vi "Weather Parse Test.vi"() -> ()   [LabVIEW 2020, in "CDM-Config.lvlib"] (continued)
             \"CMAS\"\n                    ],\n                    \"VTEC\": [\n                        \"/O.CON.KBUF.SC.Y.0098.251203T1200Z-251205T0300Z/\"\n                    ],\n                    \"eventEndingTime\": [\n                        \"2025-12-04T22:00:00-05:00\"\n                    ]\n                },\n                \"scope\": \"Public\",\n                \"code\": \"IPAWSv1.0\",\n                \"language\": \"en-US\",\n                \"web\": \"http://www.weather.gov\",\n                \"eventCode\": {\n                    \"SAME\": [\n                        \"NWS\"\n                    ],\n                    \"NationalWeatherService\": [\n                        \"SCY\"\n                    ]\n                }\n            }\n        },\n        {\n            \"id\": \"https://api.weather.gov/alerts/urn:oid:2.49.0.1.840.0.c02a5c0c1925cdd5918687c0525e8f8235dbd8da.001.1\",\n            \"type\": \"Feature\",\n            \"geometry\": null,\n            \"properties\": {\n                \"@id\": \"https://api.weather.gov/alerts/urn:oid:2.49.0.1.840.0.c02a5c0c1925cdd5918687c0525e8f8235dbd8da.001.1\",\n                \"@type\": \"wx:Alert\",\n                \"id\": \"urn:oid:2.49.0.1.840.0.c02a5c0c1925cdd5918687c0525e8f8235dbd8da.001.1\",\n                \"areaDesc\": \"Alger; Luce; Northern Schoolcraft\",\n                \"geocode\": {\n                    \"SAME\": [\n                        \"026003\",\n                        \"026095\",\n                        \"026153\"\n                    ],\n                    \"UGC\": [\n                        \"MIZ006\",\n                        \"MIZ007\",\n                        \"MIZ085\"\n                    ]\n                },\n                \"affectedZones\": [\n                    \"https://api.weather.gov/zones/forecast/MIZ006\",\n                    \"https://api.weather.gov/zones/forecast/MIZ007\",\n                    \"https://api.weather.gov/zones/forecast/MIZ085\"\n                ],\n                \"references\": [],\n                \"sent\": \"2025-12-03T03:02:00-05:00\",\n                \"effective\": \"2025-12-03T03:02:00-05:00\",\n                \"onset\": \"2025-12-03T07:00:00-05:00\",\n                \"expires\": \"2025-12-03T16:15:00-05:00\",\n                \"ends\": \"2025-12-04T07:00:00-05:00\",\n                \"status\": \"Actual\",\n                \"messageType\": \"Alert\",\n                \"category\": \"Met\",\n                \"severity\": \"Moderate\",\n                \"certainty\": \"Likely\",\n                \"urgency\": \"Expected\",\n                \"event\": \"Winter Weather Advisory\",\n                \"sender\": \"w-nws.webmaster@noaa.gov\",\n                \"senderName\": \"NWS Marquette MI\",\n                \"headline\": \"Winter Weather Advisory issued December 3 at 3:02AM EST until December 4 at 7:00AM EST by NWS Marquette MI\",\n                \"description\": \"* WHAT...Lake effect snow expected. Total snow accumulations between\\n3 and 7 inches. Winds gusting as high as 35 mph, highest along the\\nLake Superior shores.\\n\\n* WHERE...Alger, Luce, and Northern Schoolcraft Counties.\\n\\n* WHEN...From 7 AM this morning to 7 AM EST Thursday.\\n\\n* IMPACTS...Travel could be difficult. Areas of blowing snow could\\nsignificantly reduce visibility. The hazardous conditions could\\nimpact the Wednesday morning and evening commutes.\\n\\n* ADDITIONAL DETAILS...The southwest portions of Alger County such\\nas Chatham and Trenary will see snow accumulations of 2 inches or\\nless.\",\n                \"instruction\": \"Slow down and use caution while traveling.\\n\\nDuring lake effect snow, the weather can vary from bands of locally\\nheavy snow to dry weather just a few miles away. Visibilities can\\nalso vary greatly. Be prepared for rapid changes in weather,\\nvisibility, and road conditions.\",\n                \"response\": \"Execute\",\n                \"parameters\": {\n                    \"AWIPSidentifier\": [\n                        \"WSWMQT\"\n                    ],\n                    \"WMOidentifier\": [\n                        \"WWUS43 KMQT 030802\"\n                    ],\n                    \"NWSheadline\": [\n                        \"WINTER WEATHER ADVISORY IN EFFECT FROM 7 AM THIS MORNING TO 7 AM EST THURSDAY\"\n                    ],\n                    \"BLOCKCHANNEL\": [\n                        \"EAS\",\n                        \"NWEM\",\n                        \"CMAS\"\n                    ],\n                    \"VTEC\": [\n                        \"/O.NEW.KMQT.WW.Y.0035.251203T1200Z-251204T1200Z/\"\n                    ],\n                    \"eventEndingTime\": [\n                        \"2025-12-04T07:00:00-05:00\"\n                    ]\n                },\n                \"scope\": \"Public\",\n                \"code\": \"IPAWSv1.0\",\n                \"language\": \"en-US\",\n                \"web\": \"http://www.weather.gov\",\n                \"eventCode\": {\n                    \"SAME\": [\n                        \"NWS\"\n                    ],\n                    \"NationalWeatherService\": [\n                        \"WWY\"\n                    ]\n                }\n            }\n        },\n        {\n            \"id\": \"https://api.weather.gov/alerts/urn:oid:2.49.0.1.840.0.59f7e1922117cec0abab2205c7453e67e9856636.002.1\",\n            \"type\": \"Feature\",\n            \"geometry\": null,\n            \"properties\": {\n                \"@id\": \"https://api.weather.gov/alerts/urn:oid:2.49.0.1.840.0.59f7e1922117cec0abab2205c7453e67e9856636.002.1\",\n                \"@type\": \"wx:Alert\",\n                \"id\": \"urn:oid:2.49.0.1.840.0.59f7e1922117cec0abab2205c7453e67e9856636.002.1\",\n                \"areaDesc\": \"Sierra Madre Range; Snowy Range\",\n                \"geocode\": {\n                    \"SAME\": [\n                        \"056007\",\n                        \"056001\"\n                    ],\n                    \"UGC\": [\n                        \"WYZ112\",\n                        \"WYZ114\"\n                    ]\n                },\n                \"affectedZones\": [\n                    \"https://api.weather.gov/zones/forecast/WYZ112\",\n                    \"https://api.weather.gov/zones/forecast/WYZ114\"\n                ],\n                \"references\": [\n                    {\n                        \"@id\": \"https://api.weather.gov/alerts/urn:oid:2.49.0.1.840.0.87fb13f6ba1b004b93c1e82c033f30d580049308.002.1\",\n                        \"identifier\": \"urn:oid:2.49.0.1.840.0.87fb13f6ba1b004b93c1e82c033f30d580049308.002.1\",\n                        \"sender\": \"w-nws.webmaster@noaa.gov\",\n                        \"sent\": \"2025-12-02T14:13:00-07:00\"\n                    }\n                ],\n                \"sent\": \"2025-12-02T23:52:00-07:00\",\n                \"effective\": \"2025-12-02T23:52:00-07:00\",\n                \"onset\": \"2025-12-02T23:52:00-07:00\",\n                \"expires\": \"2025-12-03T11:00:00-07:00\",\n                \"ends\": \"2025-12-03T11:00:00-07:00\",\n                \"status\": \"Actual\",\n                \"messageType\": \"Update\",\n                \"category\": \"Met\",\n                \"severity\": \"Moderate\",\n                \"certainty\": \"Likely\",\n                \"urgency\": \"Expected\",\n                \"event\": \"Winter Weather Advisory\",\n                \"sender\": \"w-nws.webmaster@noaa.gov\",\n                \"senderName\": \"NWS Cheyenne WY\",\n                \"headline\": \"Winter Weather Advisory issued December 2 at 11:52PM MST until December 3 at 11:00AM MST by NWS Cheyenne WY\",\n                \"description\": \"* WHAT...Snow. Additional snow accumulations up to 3 inches.\\n\\n* WHERE...Sierra Madre Range and Snowy Range.\\n\\n* WHEN...Until 11 AM MST Wednesday.\\n\\n* IMPACTS...Outdoor recreation could become dangerous to those\\ncaught unprepared for hazardous winter conditions. Hunters,\\nhikers, and snowmobilers may become disoriented and lost due to\\nlow visibility in falling and blowing snow. Travel could be very\\ndifficult.\",\n                \"instruction\": \"Slow down and use caution while traveling. The latest road\\nconditions for the state you are calling from can be obtained by\\ncalling 5 1 1.\",\n                \"response\": \"Execute\",\n                \"parameters\": {\n                    \"AWIPSidentifier\": [\n                        \"WSWCYS\"\n                    ],\n                    \"WMOidentifier\": [\n                        \"WWUS45 KCYS 030652\"\n                    ],\n                    \"NWSheadline\": [\n                        \"WINTER WEATHER ADVISORY REMAINS IN EFFECT UNTIL 11 AM MST WEDNESDAY\"\n                    ],\n                    \"BLOCKCHANNEL\": [\n                        \"EAS\",\n                        \"NWEM\",\n                        \"CMAS\"\n                    ],\n                    \"VTEC\": [\n                        \"/O.CON.KCYS.WW.Y.0035.000000T0000Z-251203T1800Z/\"\n                    ],\n                    \"eventEndingTime\": [\n                        \"2025-12-03T11:00:00-07:00\"\n                    ],\n                    \"expiredReferences\": [\n                        \"w-nws.webmaster@noaa.gov,urn:oid:2.49.0.1.840.0.fecf578d7cc004b2e9035df7c924d23aa49b7b6f.001.1,2025-12-02T02:18:00-07:00 w-nws.webmaster@noaa.gov,urn:oid:2.49.0.1.840.0.569ad64d3405614b0a2aabc3905b3b5007dab878.001.1,2025-12-01T14:15:00-07:00 w-nws.webmaster@noaa.gov,urn:oid:2.49.0.1.840.0.9d0e156dd967b121facde90ef95bedbde49aa40d.001.1,2025-12-01T14:12:00-07:00\"\n                    ]\n                },\n                \"scope\": \"Public\",\n                \"code\": \"IPAWSv1.0\",\n                \"language\": \"en-US\",\n                \"web\": \"http://www.weather.gov\",\n                \"eventCode\": {\n                    \"SAME\": [\n                        \"NWS\"\n                    ],\n                    \"NationalWeatherService\": [\n                        \"WWY\"\n                    ]\n                }\n            }\n        },\n        {\n            \"id\": \"https://api.weather.gov/alerts/urn:oid:2.49.0.1.840.0.59f7e1922117cec0abab2205c7453e67e9856636.001.1\",\n            \"type\": \"Feature\",\n            \"geometry\": null,\n            \"properties\": {\n                \"@id\": \"https://api.weather.gov/alerts/urn:oid:2.49.0.1.840.0.59f7e1922117cec0abab2205c7453e67e9856636.001.1\",\n                \"@type\": \"wx:Alert\",\n                \"id\": \"urn:oid:2.49.0.1.840.0.59f7e1922117cec0abab2205c7453e67e9856636.001.1\",\n                \"areaDesc\": \"North Snowy Range Foothills; South Laramie Range\",\n                \"geocode\": {\n                    \"SAME\": [\n                        \"056001\",\n                        \"056007\",\n                        \"056021\"\n                    ],\n                    \"UGC\": [\n                        \"WYZ110\",\n                        \"WYZ116\"\n                    ]\n                },\n                \"affectedZones\": [\n                    \"https://api.weather.gov/zones/forecast/WYZ110\",\n                    \"https://api.weather.gov/zones/forecast/WYZ116\"\n                ],\n                \"references\": [\n                    {\n                        \"@id\": \"https://api.weather.gov/alerts/urn:oid:2.49.0.1.840.0.87fb13f6ba1b004b93c1e82c033f30d580049308.001.1\",\n                        \"identifier\": \"urn:oid:2.49.0.1.840.0.87fb13f6ba1b004b93c1e82c033f30d580049308.001.1\",\n                        \"sender\": \"w-nws.webmaster@noaa.gov\",\n                        \"sent\": \"2025-12-02T14:13:00-07:00\"\n                    }\n                ],\n                \"sent\": \"2025-12-02T23:52:00-07:00\",\n                \"effective\": \"2025-12-02T23:52:00-07:00\",\n                \"onset\": \"2025-12-02T23:52:00-07:00\",\n                \"expires\": \"2025-12-03T11:00:00-07:00\",\n                \"ends\": \"2025-12-03T11:00:00-07:00\",\n                \"status\": \"Actual\",\n                \"messageType\": \"Update\",\n                \"category\": \"Met\",\n                \"severity\": \"Moderate\",\n                \"certainty\": \"Likely\",\n                \"urgency\": \"Expected\",\n                \"event\": \"Winter Weather Advisory\",\n                \"sender\": \"w-nws.webmaster@noaa.gov\",\n                \"senderName\": \"NWS Cheyenne WY\",\n                \"headline\": \"Winter Weather Advisory issued December 2 at 11:52PM MST until December 3 at 11:00AM MST by NWS Cheyenne WY\",\n                \"description\": \"* WHAT...Snow. Additional snow accumulations up to two inches.\\n\\n* WHERE...South Laramie Range including the Interstate 80 Summit\\nbetween Cheyenne and Laramie, and North Snowy Range Foothills\\nincluding Arlington and Elk Mountain along Interstate 80.\\n\\n* WHEN...Until 11 AM MST Wednesday.\\n\\n* IMPACTS...Plan on slippery road conditions. The hazardous\\nconditions could impact the Wednesday morning commute.\",\n                \"instruction\": \"Slow down and use caution while traveling. The latest road\\nconditions for the state you are calling from can be obtained by\\ncalling 5 1 1.\",\n                \"response\": \"Execute\",\n                \"parameters\": {\n                    \"AWIPSidentifier\": [\n                        \"WSWCYS\"\n                    ],\n                    \"WMOidentifier\": [\n                        \"WWUS45 KCYS 030652\"\n                    ],\n                    \"NWSheadline\": [\n                        \"WINTER WEATHER ADVISORY REMAINS IN EFFECT UNTIL 11 AM MST WEDNESDAY\"\n                    ],\n                    \"BLOCKCHANNEL\": [\n                        \"EAS\",\n                        \"NWEM\",\n                        \"CMAS\"\n                    ],\n                    \"VTEC\": [\n                        \"/O.CON.KCYS.WW.Y.0035.000000T0000Z-251203T1800Z/\"\n                    ],\n                    \"eventEndingTime\": [\n                        \"2025-12-03T11:00:00-07:00\"\n                    ]\n                },\n                \"scope\": \"Public\",\n                \"code\": \"IPAWSv1.0\",\n                \"language\": \"en-US\",\n                \"web\": \"http://www.weather.gov\",\n                \"eventCode\": {\n                    \"SAME\": [\n                        \"NWS\"\n                    ],\n                    \"NationalWeatherService\": [\n                        \"WWY\"\n                    ]\n                }\n            }\n        },\n        {\n            \"id\": \"https://api.weather.gov/alerts/urn:oid:2.49.0.1.840.0.f60d42f0491b4e02db9492f5ccb8a64bf6617900.001.1\",\n            \"type\": \"Feature\",\n            \"geometry\": null,\n            \"properties\": {\n                \"@id\": \"https://api.weather.gov/alerts/urn:oid:2.49.0.1.840.0.f60d42f0491b4e02db9492f5ccb8a64bf6617900.001.1\",\n                \"@type\": \"wx:Alert\",\n                \"id\": \"urn:oid:2.49.0.1.840.0.f60d42f0491b4e02db9492f5ccb8a64bf6617900.001.1\",\n                \"areaDesc\": \"Chuuk Lagoon\",\n                \"geocode\": {\n                    \"SAME\": [\n                        \"064002\"\n                    ],\n                    \"UGC\": [\n                        \"FMZ023\"\n                    ]\n                },\n                \"affectedZones\": [\n                    \"https://api.weather.gov/zones/forecast/FMZ023\"\n                ],\n                \"references\": [],\n                \"sent\": \"2025-12-03T16:48:00+10:00\",\n                \"effective\": \"2025-12-03T16:48:00+10:00\",\n                \"onset\": \"2025-12-04T17:00:00+10:00\",\n                \"expires\": \"2025-12-04T07:00:00+10:00\",\n                \"ends\": \"2025-12-06T17:00:00+10:00\",\n                \"status\": \"Actual\",\n                \"messageType\": \"Alert\",\n                \"category\": \"Met\",\n                \"severity\": \"Minor\",\n                \"certainty\": \"Likely\",\n                \"urgency\": \"Expected\",\n                \"event\": \"Coastal Flood Advisory\",\n                \"sender\": \"w-nws.webmaster@noaa.gov\",\n                \"senderName\": \"NWS Tiyan GU\",\n                \"headline\": \"Coastal Flood Advisory issued December 3 at 4:48PM ChST until December 6 at 5:00PM ChST by NWS Tiyan GU\",\n                \"description\": \"* WHAT...Minor coastal flooding expected.\\n\\n* WHERE...North and east facing reefs of Chuuk.\\n\\n* WHEN...From 5 PM Thursday to 5 PM ChST Saturday.\\n\\n* IMPACTS...Flooding of lots, parks, and roads with only isolated\\nroad closures expected.\\n\\n* ADDITIONAL DETAILS...A long-period north swell combined with above\\nnortmal King Tides will produce minor coastal flooding during high\\ntide Thursday afternoon into the weekend. If the north swell\\nremains longer than expected, flooding could continue into Sunday.\\nHigh tides will begin to decrease Sunday afternoon.\",\n                \"instruction\": \"A coastal flood advisory indicates that onshore winds and tides\\nwill combine to generate flooding of low areas along the shore.\\n\\nWatch for debris along low-lying shorelines facing north and\\neast. Residents living along these low-lying shorelines need to\\nmonitor water levels and take actions to protect property from\\ninundation.\",\n                \"response\": \"Monitor\",\n                \"parameters\": {\n                    \"AWIPSidentifier\": [\n                        \"CFWPQ2\"\n                    ],\n                    \"WMOidentifier\": [\n                        \"WHPQ42 PGUM 030648\"\n                    ],\n                    \"NWSheadline\": [\n                        \"COASTAL FLOOD ADVISORY IN EFFECT FROM 5 PM THURSDAY TO 5 PM CHST SATURDAY\"\n                    ],\n                    \"BLOCKCHANNEL\": [\n                        \"EAS\",\n                        \"NWEM\",\n                        \"CMAS\"\n                    ],\n                    \"VTEC\": [\n                        \"/O.NEW.PGUM.CF.Y.0005.251204T0700Z-251206T0700Z/\"\n                    ],\n                    \"eventEndingTime\": [\n                        \"2025-12-06T17:00:00+10:00\"\n                    ]\n                },\n                \"scope\": \"Public\",\n                \"code\": \"IPAWSv1.0\",\n                \"language\": \"en-US\",\n                \"web\": \"http://www.weather.gov\",\n                \"eventCode\": {\n                    \"SAME\": [\n                        \"NWS\"\n                    ],\n                    \"NationalWeatherService\": [\n                        \"CFY\"\n                    ]\n                }\n            }\n        },\n        {\n            \"id\": \"https://api.weather.gov/alerts/urn:oid:2.49.0.1.840.0.494bb19814f8e44e3444f0a72cb5e83723369712.004.1\",\n            \"type\": \"Feature\",\n            \"geometry\": null,\n            \"properties\": {\n                \"@id\": \"https://api.weather.gov/alerts/urn:oid:2.49.0.1.840.0.494bb19814f8e44e3444f0a72cb5e83723369712.004.1\",\n                \"@type\": \"wx:Alert\",\n                \"id\": \"urn:oid:2.49.0.1.840.0.494bb19814f8e44e3444f0a72cb5e83723369712.004.1\",\n                \"areaDesc\": \"Western Santa Monica Mountains Recreational Area; Eastern Santa Monica Mountains Recreational Area; Santa Susana Mountains; Southern Ventura County Mountains; Interstate 5 Corridor; Western San Gabriel Mountains and Highway 14 Corridor; Eastern San Gabriel Mountains\",\n                \"geocode\": {\n                    \"SAME\": [\n                        \"006037\",\n                        \"006111\"\n                    ],\n                    \"UGC\": [\n                        \"CAZ369\",\n                        \"CAZ370\",\n                        \"CAZ375\",\n                        \"CAZ376\",\n                        \"CAZ378\",\n                        \"CAZ379\",\n                        \"CAZ380\"\n                    ]\n                },\n                \"affectedZones\": [\n                    \"https://api.weather.gov/zones/forecast/CAZ369\",\n                    \"https://api.weather.gov/zones/forecast/CAZ370\",\n                    \"https://api.weather.gov/zones/forecast/CAZ375\",\n                    \"https://api.weather.gov/zones/forecast/CAZ376\",\n                    \"https://api.weather.gov/zones/forecast/CAZ378\",\n                    \"https://api.weather.gov/zones/forecast/CAZ379\",\n                    \"https://api.weather.gov/zones/forecast/CAZ380\"\n                ],\n                \"references\": [\n                    {\n                        \"@id\": \"https://api.weather.gov/alerts/urn:oid:2.49.0.1.840.0.689b4595aa089b11e65682ac050dc73cf4aaa636.002.1\",\n                        \"identifier\": \"urn:oid:2.49.0.1.840.0.689b4595aa089b11e65682ac050dc73cf4aaa636.002.1\",\n                        \"sender\": \"w-nws.webmaster@noaa.gov\",\n                        \"sent\": \"2025-12-02T10:40:00-08:00\"\n                    },\n                    {\n                        \"@id\": \"https://api.weather.gov/alerts/urn:oid:2.49.0.1.840.0.0d5a73fd09523b91e12026c87a917b096083ea16.003.1\",\n                        \"identifier\": \"urn:oid:2.49.0.1.840.0.0d5a73fd09523b91e12026c87a917b096083ea16.003.1\",\n                        \"sender\": \"w-nws.webmaster@noaa.gov\",\n                        \"sent\": \"2025-12-02T12:01:00-08:00\"\n                    },\n                    {\n                        \"@id\": \"https://api.weather.gov/alerts/urn:oid:2.49.0.1.840.0.6cc491b4db559442d77c3eb01f79e9eafe0c07db.004.1\",\n                        \"identifier\": \"urn:oid:2.49.0.1.840.0.6cc491b4db559442d77c3eb01f79e9eafe0c07db.004.1\",\n                        \"sender\": \"w-nws.webmaster@noaa.gov\",\n                        \"sent\": \"2025-12-02T14:21:00-08:00\"\n                    }\n                ],\n                \"sent\": \"2025-12-02T22:45:00-08:00\",\n                \"effective\": \"2025-12-02T22:45:00-08:00\",\n                \"onset\": \"2025-12-03T06:00:00-08:00\",\n                \"expires\": \"2025-12-03T08:00:00-08:00\",\n                \"ends\": \"2025-12-04T15:00:00-08:00\",\n                \"status\": \"Actual\",\n                \"messageType\": \"Update\",\n                \"category\": \"Met\",\n                \"severity\": \"Moderate\",\n                \"certainty\": \"Likely\",\n                \"urgency\": \"Expected\",\n                \"event\": \"Wind Advisory\",\n                \"sender\": \"w-nws.webmaster@noaa.gov\",\n                \"senderName\": \"NWS Los Angeles/Oxnard CA\",\n                \"headline\": \"Wind Advisory issued December 2 at 10:45PM PST until December 4 at 3:00PM PST by NWS Los Angeles/Oxnard CA\",\n                \"description\": \"* WHAT...Northeast winds 25 to 40 mph with gusts of 40 to 55 mph\\nexpected. Isolated gusts to 60 mph are possible.\\n\\n* WHERE...Eastern San Gabriel Mountains, Eastern Santa Monica\\nMountains Recreational Area, Interstate 5 Corridor, Santa Susana\\nMountains, Southern Ventura County Mountains, Western San Gabriel\\nMountains and Highway 14 Corridor, and Western Santa Monica\\nMountains Recreational Area.\\n\\n* WHEN...From 6 AM Wednesday to 3 PM PST Thursday.\\n\\n* IMPACTS...Gusty winds will blow around unsecured objects. Tree\\nlimbs could be blown down and a few power outages may result.\\nEntire trees may also be blown over more easily due to wet soils\\nfrom the November rains.\\n\\n* ADDITIONAL DETAILS...Relative lulls are possible in the late\\nafternoon through evening hours Wednesday.\",\n                \"instruction\": \"Winds this strong can make driving difficult, especially for high\\nprofile vehicles. Use extra caution. Be cautious parking under trees.\",\n                \"response\": \"Execute\",\n                \"parameters\": {\n                    \"AWIPSidentifier\": [\n                        \"NPWLOX\"\n                    ],\n                    \"WMOidentifier\": [\n                        \"WWUS76 KLOX 030645\"\n                    ],\n                    \"NWSheadline\": [\n                        \"WIND ADVISORY REMAINS IN EFFECT FROM 6 AM WEDNESDAY TO 3 PM PST THURSDAY\"\n                    ],\n                    \"BLOCKCHANNEL\": [\n                        \"EAS\",\n                        \"NWEM\",\n                        \"CMAS\"\n                    ],\n                    \"VTEC\": [\n                        \"/O.CON.KLOX.WI.Y.0091.251203T1400Z-251204T2300Z/\"\n                    ],\n                    \"eventEndingTime\": [\n                        \"2025-12-04T15:00:00-08:00\"\n                    ]\n                },\n                \"scope\": \"Public\",\n                \"code\": \"IPAWSv1.0\",\n                \"language\": \"en-US\",\n                \"web\": \"http://www.weather.gov\",\n                \"eventCode\": {\n                    \"SAME\": [\n                        \"NWS\"\n                    ],\n                    \"NationalWeatherService\": [\n                        \"WIY\"\n                    ]\n                }\n            }\n        },\n        {\n            \"id\": \"https://api.weather.gov/alerts/urn:oid:2.49.0.1.840.0.494bb19814f8e44e3444f0a72cb5e83723369712.003.1\",\n            \"type\": \"Feature\",\n            \"geometry\": null,\n            \"properties\": {\n                \"@id\": \"https://api.weather.gov/alerts/urn:oid:2.49.0.1.840.0.494bb19814f8e44e3444f0a72cb5e83723369712.003.1\",\n                \"@type\": \"wx:Alert\",\n                \"id\": \"urn:oid:2.49.0.1.840.0.494bb19814f8e44e3444f0a72cb5e83723369712.003.1\",\n                \"areaDesc\": \"Santa Clarita Valley; Ventura County Beaches; Ventura County Inland Coast; Central Ventura County Valleys; Malibu Coast; Calabasas and Agoura Hills; Southeastern Ventura County Valleys\",\n                \"geocode\": {\n                    \"SAME\": [\n                        \"006037\",\n                        \"006111\"\n                    ],\n                    \"UGC\": [\n                        \"CAZ088\",\n                        \"CAZ354\",\n                        \"CAZ355\",\n                        \"CAZ358\",\n                        \"CAZ362\",\n                        \"CAZ371\",\n                        \"CAZ374\"\n                    ]\n                },\n                \"affectedZones\": [\n                    \"https://api.weather.gov/zones/forecast/CAZ088\",\n                    \"https://api.weather.gov/zones/forecast/CAZ354\",\n                    \"https://api.weather.gov/zones/forecast/CAZ355\",\n                    \"https://api.weather.gov/zones/forecast/CAZ358\",\n                    \"https://api.weather.gov/zones/forecast/CAZ362\",\n                    \"https://api.weather.gov/zones/forecast/CAZ371\",\n                    \"https://api.weather.gov/zones/forecast/CAZ374\"\n                ],\n                \"references\": [\n                    {\n                        \"@id\": \"https://api.weather.gov/alerts/urn:oid:2.49.0.1.840.0.689b4595aa089b11e65682ac050dc73cf4aaa636.001.1\",\n                        \"identifier\": \"urn:oid:2.49.0.1.840.0.689b4595aa089b11e65682ac050dc73cf4aaa636.001.1\",\n                        \"sender\": \"w-nws.webmaster@noaa.gov\",\n                        \"sent\": \"2025-12-02T10:40:00-08:00\"\n                    },\n                    {\n                        \"@id\": \"https://api.weather.gov/alerts/urn:oid:2.49.0.1.840.0.0d5a73fd09523b91e12026c87a917b096083ea16.002.1\",\n                        \"identifier\": \"urn:oid:2.49.0.1.840.0.0d5a73fd09523b91e12026c87a917b096083ea16.002.1\",\n                        \"sender\": \"w-nws.webmaster@noaa.gov\",\n                        \"sent\": \"2025-12-02T12:01:00-08:00\"\n                    },\n                    {\n                        \"@id\": \"https://api.weather.gov/alerts/urn:oid:2.49.0.1.840.0.6cc491b4db559442d77c3eb01f79e9eafe0c07db.003.1\",\n                        \"identifier\": \"urn:oid:2.49.0.1.840.0.6cc491b4db559442d77c3eb01f79e9eafe0c07db.003.1\",\n                        \"sender\": \"w-nws.webmaster@noaa.gov\",\n                        \"sent\": \"2025-12-02T14:21:00-08:00\"\n                    }\n                ],\n                \"sent\": \"2025-12-02T22:45:00-08:00\",\n                \"effective\": \"2025-12-02T22:45:00-08:00\",\n                \"onset\": \"2025-12-03T06:00:00-08:00\",\n                \"expires\": \"2025-12-03T08:00:00-08:00\",\n                \"ends\": \"2025-12-04T15:00:00-08:00\",\n                \"status\": \"Actual\",\n                \"messageType\": \"Update\",\n                \"category\": \"Met\",\n                \"severity\": \"Moderate\",\n                \"certainty\": \"Likely\",\n                \"urgency\": \"Expected\",\n                \"event\": \"Wind Advisory\",\n                \"sender\": \"w-nws.webmaster@noaa.gov\",\n                \"senderName\": \"NWS Los Angeles/Oxnard CA\",\n                \"headline\": \"Wind Advisory issued December 2 at 10:45PM PST until December 4 at 3:00PM PST by NWS Los Angeles/Oxnard CA\",\n                \"description\": \"* WHAT...Northeast gusts 25 to 35 mph, with local areas gusting up\\nto 45 mph in favored foothills.\\n\\n* WHERE...Calabasas and Agoura Hills, Central Ventura County\\nValleys, Malibu Coast, Santa Clarita Valley, Southeastern Ventura\\nCounty Valleys, Ventura County Beaches, and Ventura County Inland\\nCoast.\\n\\n* WHEN...From 6 AM Wednesday to 3 PM PST Thursday.\\n\\n* IMPACTS...Gusty winds will blow around unsecured objects. Tree\\nlimbs could be blown down and a few power outages may result.\\nEntire trees may also be blown over more easily due to wet soils\\nfrom from the November rains.\\n\\n* ADDITIONAL DETAILS...Relative lulls are possible in the late\\nafternoon through evening hours Wednesday.\",\n                \"instruction\": \"Winds this strong can make driving difficult, especially for high\\nprofile vehicles. Be cautious parking under trees. Secure outdoor\\nobjects.\",\n                \"response\": \"Execute\",\n                \"parameters\": {\n                    \"AWIPSidentifier\": [\n                        \"NPWLOX\"\n                    ],\n                    \"WMOidentifier\": [\n                        \"WWUS76 KLOX 030645\"\n                    ],\n                    \"NWSheadline\": [\n                        \"WIND ADVISORY REMAINS IN EFFECT FROM 6 AM WEDNESDAY TO 3 PM PST THURSDAY\"\n                    ],\n                    \"BLOCKCHANNEL\": [\n                        \"EAS\",\n                        \"NWEM\",\n                        \"CMAS\"\n                    ],\n                    \"VTEC\": [\n                        \"/O.CON.KLOX.WI.Y.0091.251203T1400Z-251204T2300Z/\"\n                    ],\n                    \"eventEndingTime\": [\n                        \"2025-12-04T15:00:00-08:00\"\n                    ]\n                },\n                \"scope\": \"Public\",\n                \"code\": \"IPAWSv1.0\",\n                \"language\": \"en-US\",\n                \"web\": \"http://www.weather.gov\",\n                \"eventCode\": {\n                    \"SAME\": [\n                        \"NWS\"\n                    ],\n                    \"NationalWeatherService\": [\n                        \"WIY\"\n                    ]\n                }\n            }\n        },\n        {\n            \"id\": \"https://api.weather.gov/alerts/urn:oid:2.49.0.1.840.0.73842cfd87f41127d31e81fcc67d03a233033278.002.1\",\n            \"type\": \"Feature\",\n            \"geometry\": null,\n            \"properties\": {\n                \"@id\": \"https://api.weather.gov/alerts/urn:oid:2.49.0.1.840.0.73842cfd87f41127d31e81fcc67d03a233033278.002.1\",\n                \"@type\": \"wx:Alert\",\n                \"id\": \"urn:oid:2.49.0.1.840.0.73842cfd87f41127d31e81fcc67d03a233033278.002.1\",\n                \"areaDesc\": \"Waters from Cape Blanco OR to Pt. St. George CA from 10 to 60 nm\",\n                \"geocode\": {\n                    \"SAME\": [\n                        \"057376\"\n                    ],\n                    \"UGC\": [\n                        \"PZZ376\"\n                    ]\n                },\n                \"affectedZones\": [\n                    \"https://api.weather.gov/zones/forecast/PZZ376\"\n                ],\n                \"references\": [\n                    {\n                        \"@id\": \"https://api.weather.gov/alerts/urn:oid:2.49.0.1.840.0.ff4bbfd20da4fd1cce1c220878d6bd0da88828d2.002.1\",\n                        \"identifier\": \"urn:oid:2.49.0.1.840.0.ff4bbfd20da4fd1cce1c220878d6bd0da88828d2.002.1\",\n                        \"sender\": \"w-nws.webmaster@noaa.gov\",\n                        \"sent\": \"2025-12-02T11:28:00-08:00\"\n                    }\n                ],\n                \"sent\": \"2025-12-02T22:30:00-08:00\",\n                \"effective\": \"2025-12-02T22:30:00-08:00\",\n                \"onset\": \"2025-12-02T22:30:00-08:00\",\n                \"expires\": \"2025-12-03T14:00:00-08:00\",\n                \"ends\": \"2025-12-04T10:00:00-08:00\",\n                \"status\": \"Actual\",\n                \"messageType\": \"Update\",\n                \"category\": \"Met\",\n                \"severity\": \"Minor\",\n                \"certainty\": \"Likely\",\n                \"urgency\": \"Expected\",\n                \"event\": \"Small Craft Advisory\",\n                \"sender\": \"w-nws.webmaster@noaa.gov\",\n                \"senderName\": \"NWS Medford OR\",\n                \"headline\": \"Small Craft Advisory issued December 2 at 10:30PM PST until December 4 at 10:00AM PST by NWS Medford OR\",\n                \"description\": \"* WHAT...North winds 15 to 25 kt with gusts up to 30 kt and steep\\nseas 6 to 11 ft due to long period northwest swell and wind\\nwaves.\\n\\n* WHERE...South of Port Orford.\\n\\n* WHEN...Until 10 AM PST Thursday.\\n\\n* IMPACTS...Gusty winds and/or steep seas could capsize or\\ndamage smaller vessels.\\n\\n* View the hazard area in detail at https://go.usa.gov/x6hks\",\n                \"instruction\": \"Inexperienced mariners and those operating smaller vessels should\\nremain in port and avoid the area of hazardous conditions.\",\n                \"response\": \"Avoid\",\n                \"parameters\": {\n                    \"AWIPSidentifier\": [\n                        \"MWWMFR\"\n                    ],\n                    \"WMOidentifier\": [\n                        \"WHUS76 KMFR 030630\"\n                    ],\n                    \"NWSheadline\": [\n                        \"SMALL CRAFT ADVISORY REMAINS IN EFFECT UNTIL 10 AM PST THURSDAY\"\n                    ],\n                    \"BLOCKCHANNEL\": [\n                        \"EAS\",\n                        \"NWEM\",\n                        \"CMAS\"\n                    ],\n                    \"VTEC\": [\n                        \"/O.CON.KMFR.SC.Y.0105.000000T0000Z-251204T1800Z/\"\n                    ],\n                    \"eventEndingTime\": [\n                        \"2025-12-04T10:00:00-08:00\"\n                    ],\n                    \"expiredReferences\": [\n                        \"w-nws.webmaster@noaa.gov,urn:oid:2.49.0.1.840.0.9ce8ff0ba6cf0f16fd881abc502d3d38578d9b04.002.1,2025-12-02T06:58:00-08:00 w-nws.webmaster@noaa.gov,urn:oid:2.49.0.1.840.0.100cb0978a3599b33dbb2831cbb857a24fe9f087.002.1,2025-12-01T14:14:00-08:00 w-nws.webmaster@noaa.gov,urn:oid:2.49.0.1.840.0.683735be588e5c6cd6552754ce0abe986105e8f4.002.1,2025-12-01T08:09:00-08:00 w-nws.webmaster@noaa.gov,urn:oid:2.49.0.1.840.0.dc099e3376272b5fd3a4f51e00bf8256c7349df9.002.1,2025-11-30T14:09:00-08:00 w-nws.webmaster@noaa.gov,urn:oid:2.49.0.1.840.0.f1d7a7cf4acbda0839d8e3a995234e56c06b660e.002.1,2025-11-30T03:18:00-08:00 w-nws.webmaster@noaa.gov,urn:oid:2.49.0.1.840.0.0203c05339a024f86b055f1b0c2ab8cb1810bd96.001.1,2025-11-29T12:23:00-08:00\"\n                    ]\n                },\n                \"scope\": \"Public\",\n                \"code\": \"IPAWSv1.0\",\n                \"language\": \"en-US\",\n                \"web\": \"http://www.weather.gov\",\n                \"eventCode\": {\n                    \"SAME\": [\n                        \"NWS\"\n                    ],\n                    \"NationalWeatherService\": [\n                        \"SCY\"\n                    ]\n                }\n            }\n        },\n        {\n            \"id\": \"https://api.weather.gov/alerts/urn:oid:2.49.0.1.840.0.73842cfd87f41127d31e81fcc67d03a233033278.001.1\",\n            \"type\": \"Feature\",\n            \"geometry\": null,\n            \"properties\": {\n                \"@id\": \"https://api.weather.gov/alerts/urn:oid:2.49.0.1.840.0.73842cfd87f41127d31e81fcc67d03a233033278.001.1\",\n                \"@type\": \"wx:Alert\",\n                \"id\": \"urn:oid:2.49.0.1.840.0.73842cfd87f41127d31e81fcc67d03a233033278.001.1\",\n                \"areaDesc\": \"Coastal waters from Cape Blanco OR to Pt. St. George CA out 10 nm\",\n                \"geocode\": {\n                    \"SAME\": [\n                        \"057356\"\n                    ],\n                    \"UGC\": [\n                        \"PZZ356\"\n                    ]\n                },\n                \"affectedZones\": [\n                    \"https://api.weather.gov/zones/forecast/PZZ356\"\n                ],\n                \"references\": [\n                    {\n                        \"@id\": \"https://api.weather.gov/alerts/urn:oid:2.49.0.1.840.0.ff4bbfd20da4fd1cce1c220878d6bd0da88828d2.001.1\",\n                        \"identifier\": \"urn:oid:2.49.0.1.840.0.ff4bbfd20da4fd1cce1c220878d6bd0da88828d2.001.1\",\n                        \"sender\": \"w-nws.webmaster@noaa.gov\",\n                        \"sent\": \"2025-12-02T11:28:00-08:00\"\n                    }\n                ],\n                \"sent\": \"2025-12-02T22:30:00-08:00\",\n                \"effective\": \"2025-12-02T22:30:00-08:00\",\n                \"onset\": \"2025-12-02T22:30:00-08:00\",\n                \"expires\": \"2025-12-03T14:00:00-08:00\",\n                \"ends\": \"2025-12-04T10:00:00-08:00\",\n                \"status\": \"Actual\",\n                \"messageType\": \"Update\",\n                \"category\": \"Met\",\n                \"severity\": \"Minor\",\n                \"certainty\": \"Likely\",\n                \"urgency\": \"Expected\",\n                \"event\": \"Small Craft Advisory\",\n                \"sender\": \"w-nws.webmaster@noaa.gov\",\n                \"senderName\": \"NWS Medford OR\",\n                \"headline\": \"Small Craft Advisory issued December 2 at 10:30PM PST until December 4 at 10:00AM PST by NWS Medford OR\",\n                \"description\": \"* WHAT...North winds 15 to 25 kt with gusts up to 30 kt and steep\\nseas 6 to 9 ft due to long period northwest swell and wind\\nwaves.\\n\\n* WHERE...Areas beyond 5 nm from shore and south of Port Orford.\\n\\n* WHEN...Until 10 AM PST Thursday.\\n\\n* IMPACTS...Gusty winds and/or steep seas could capsize or\\ndamage smaller vessels.\\n\\n* View the hazard area in detail at https://go.usa.gov/x6hks\",\n                \"instruction\": \"Inexperienced mariners and those operating smaller vessels should\\nremain in port and avoid the area of hazardous conditions.\",\n                \"response\": \"Avoid\",\n                \"parameters\": {\n                    \"AWIPSidentifier\": [\n                        \"MWWMFR\"\n                    ],\n                    \"WMOidentifier\": [\n                        \"WHUS76 KMFR 030630\"\n                    ],\n                    \"NWSheadline\": [\n                        \"SMALL CRAFT ADVISORY REMAINS IN EFFECT UNTIL 10 AM PST THURSDAY\"\n                    ],\n                    \"BLOCKCHANNEL\": [\n                        \"EAS\",\n                        \"NWEM\",\n                        \"CMAS\"\n                    ],\n                    \"VTEC\": [\n                        \"/O.CON.KMFR.SC.Y.0106.000000T0000Z-251204T1800Z/\"\n                    ],\n                    \"eventEndingTime\": [\n                        \"2025-12-04T10:00:00-08:00\"\n                    ],\n                    \"expiredReferences\": [\n                        \"w-nws.webmaster@noaa.gov,urn:oid:2.49.0.1.840.0.9ce8ff0ba6cf0f16fd881abc502d3d38578d9b04.001.1,2025-12-02T06:58:00-08:00 w-nws.webmaster@noaa.gov,urn:oid:2.49.0.1.840.0.100cb0978a3599b33dbb2831cbb857a24fe9f087.001.1,2025-12-01T14:14:00-08:00 w-nws.webmaster@noaa.gov,urn:oid:2.49.0.1.840.0.683735be588e5c6cd6552754ce0abe986105e8f4.001.1,2025-12-01T08:09:00-08:00 w-nws.webmaster@noaa.gov,urn:oid:2.49.0.1.840.0.dc099e3376272b5fd3a4f51e00bf8256c7349df9.001.2,2025-11-30T14:09:00-08:00 w-nws.webmaster@noaa.gov,urn:oid:2.49.0.1.840.0.f1d7a7cf4acbda0839d8e3a995234e56c06b660e.001.2,2025-11-30T03:18:00-08:00\"\n                    ]\n                },\n                \"scope\": \"Public\",\n                \"code\": \"IPAWSv1.0\",\n                \"language\": \"en-US\",\n                \"web\": \"http://www.weather.gov\",\n                \"eventCode\": {\n                    \"SAME\": [\n                        \"NWS\"\n                    ],\n                    \"NationalWeatherService\": [\n                        \"SCY\"\n                    ]\n                }\n            }\n        },\n        {\n            \"id\": \"https://api.weather.gov/alerts/urn:oid:2.49.0.1.840.0.754d94acb6157b7488fd0326428ea0a9a1236f3d.001.1\",\n            \"type\": \"Feature\",\n            \"geometry\": null,\n            \"properties\": {\n                \"@id\": \"https://api.weather.gov/alerts/urn:oid:2.49.0.1.840.0.754d94acb6157b7488fd0326428ea0a9a1236f3d.001.1\",\n                \"@type\": \"wx:Alert\",\n                \"id\": \"urn:oid:2.49.0.1.840.0.754d94acb6157b7488fd0326428ea0a9a1236f3d.001.1\",\n                \"areaDesc\": \"Northern Humboldt Coast\",\n                \"geocode\": {\n                    \"SAME\": [\n                        \"006023\"\n                    ],\n                    \"UGC\": [\n                        \"CAZ103\"\n                    ]\n                },\n                \"affectedZones\": [\n                    \"https://api.weather.gov/zones/forecast/CAZ103\"\n                ],\n                \"references\": [\n                    {\n                        \"@id\": \"https://api.weather.gov/alerts/urn:oid:2.49.0.1.840.0.48b666a9a788255cd85c3749f45e59ccfae17eb0.001.2\",\n                        \"identifier\": \"urn:oid:2.49.0.1.840.0.48b666a9a788255cd85c3749f45e59ccfae17eb0.001.2\",\n                        \"sender\": \"w-nws.webmaster@noaa.gov\",\n                        \"sent\": \"2025-12-02T14:32:00-08:00\"\n                    }\n                ],\n                \"sent\": \"2025-12-02T21:51:00-08:00\",\n                \"effective\": \"2025-12-02T21:51:00-08:00\",\n                \"onset\": \"2025-12-03T08:00:00-08:00\",\n                \"expires\": \"2025-12-03T11:00:00-08:00\",\n                \"ends\": \"2025-12-03T11:00:00-08:00\",\n                \"status\": \"Actual\",\n                \"messageType\": \"Update\",\n                \"category\": \"Met\",\n                \"severity\": \"Minor\",\n                \"certainty\": \"Likely\",\n                \"urgency\": \"Expected\",\n                \"event\": \"Coastal Flood Advisory\",\n                \"sender\": \"w-nws.webmaster@noaa.gov\",\n                \"senderName\": \"NWS Eureka CA\",\n                \"headline\": \"Coastal Flood Advisory issued December 2 at 9:51PM PST until December 3 at 11:00AM PST by NWS Eureka CA\",\n                \"description\": \"* WHAT...High astronomical tides will cause minor flooding in\\nlow lying areas around Humboldt Bay. Up to one half foot of\\nsaltwater inundation above ground level is possible near\\nshorelines and tidal waterways. Between 8.8 and 9.1 feet MLLW\\nat the North Spit tide gauge is predicted.\\n\\n* WHERE...Northern Humboldt Coast County.\\n\\n* WHEN...For the Coastal Flood Advisory, from 8 AM to 11 AM PST\\nWednesday. For the Beach Hazards Statement, until 3 PM PST\\nthis afternoon. High tide is at 9:23 AM at the Humboldt Bay\\nNorth Spit tide gauge. Saltwater inundation will be possible 1\\nto 2 hours before and after high tide.\\n\\n* IMPACTS...Flooding of low lying areas around Humboldt Bay\\nincluding parks and roads with only isolated closures\\nexpected. Flooding will likely impact Jackson Ranch Road in\\nthe Arcata Bottoms and several roads in King Salmon.\",\n                \"instruction\": \"A Coastal Flood Advisory indicates that onshore winds and tides\\nwill combine to generate flooding of low areas along the shore.\\n\\nFeet Above Ground is locally defined as feet above the Highest\\nAstronomical Tide or HAT.\",\n                \"response\": \"Monitor\",\n                \"parameters\": {\n                    \"AWIPSidentifier\": [\n                        \"CFWEKA\"\n                    ],\n                    \"WMOidentifier\": [\n                        \"WHUS46 KEKA 030551\"\n                    ],\n                    \"NWSheadline\": [\n                        \"COASTAL FLOOD ADVISORY REMAINS IN EFFECT FROM 8 AM TO 11 AM PST WEDNESDAY\"\n                    ],\n                    \"BLOCKCHANNEL\": [\n                        \"EAS\",\n                        \"NWEM\",\n                        \"CMAS\"\n                    ],\n                    \"VTEC\": [\n                        \"/O.CON.KEKA.CF.Y.0008.251203T1600Z-251203T1900Z/\"\n                    ],\n                    \"eventEndingTime\": [\n                        \"2025-12-03T11:00:00-08:00\"\n                    ],\n                    \"expiredReferences\": [\n                        \"w-nws.webmaster@noaa.gov,urn:oid:2.49.0.1.840.0.2608130660d067239b9f8296a08f91b3a58435d3.001.1,2025-12-02T12:14:00-08:00\"\n                    ]\n                },\n                \"scope\": \"Public\",\n                \"code\": \"IPAWSv1.0\",\n                \"language\": \"en-US\",\n                \"web\": \"http://www.weather.gov\",\n                \"eventCode\": {\n                    \"SAME\": [\n                        \"NWS\"\n                    ],\n                    \"NationalWeatherService\": [\n                        \"CFY\"\n                    ]\n                }\n            }\n        },\n        {\n            \"id\": \"https://api.weather.gov/alerts/urn:oid:2.49.0.1.840.0.f25f3139d57c0fbafce18e4394cec8e3387cc317.001.2\",\n            \"type\": \"Feature\",\n            \"geometry\": null,\n            \"properties\": {\n                \"@id\": \"https://api.weather.gov/alerts/urn:oid:2.49.0.1.840.0.f25f3139d57c0fbafce18e4394cec8e3387cc317.001.2\",\n                \"@type\": \"wx:Alert\",\n                \"id\": \"urn:oid:2.49.0.1.840.0.f25f3139d57c0fbafce18e4394cec8e3387cc317.001.2\",\n                \"areaDesc\": \"Guam; Rota; Tinian; Saipan\",\n                \"geocode\": {\n                    \"SAME\": [\n                        \"066010\",\n                        \"069100\",\n                        \"069120\",\n                        \"069110\"\n                    ],\n                    \"UGC\": [\n                        \"GUZ001\",\n                        \"MPZ001\",\n                        \"MPZ002\",\n                        \"MPZ003\"\n                    ]\n                },\n                \"affectedZones\": [\n                    \"https://api.weather.gov/zones/forecast/GUZ001\",\n                    \"https://api.weather.gov/zones/forecast/MPZ001\",\n                    \"https://api.weather.gov/zones/forecast/MPZ002\",\n                    \"https://api.weather.gov/zones/forecast/MPZ003\"\n                ],\n                \"references\": [\n                    {\n                        \"@id\": \"https://api.weather.gov/alerts/urn:oid:2.49.0.1.840.0.5c24cf00b8ce0d30ec10243f5e3d0d1b92563257.001.2\",\n                        \"identifier\": \"urn:oid:2.49.0.1.840.0.5c24cf00b8ce0d30ec10243f5e3d0d1b92563257.001.2\",\n                        \"sender\": \"w-nws.webmaster@noaa.gov\",\n                        \"sent\": \"2025-12-02T15:11:00+10:00\"\n                    },\n                    {\n                        \"@id\": \"https://api.weather.gov/alerts/urn:oid:2.49.0.1.840.0.56606cf3de3759568a567931443b4c170707798d.001.2\",\n                        \"identifier\": \"urn:oid:2.49.0.1.840.0.56606cf3de3759568a567931443b4c170707798d.001.2\",\n                        \"sender\": \"w-nws.webmaster@noaa.gov\",\n                        \"sent\": \"2025-12-03T04:02:00+10:00\"\n                    }\n                ],\n                \"sent\": \"2025-12-03T14:45:00+10:00\",\n                \"effective\": \"2025-12-03T14:45:00+10:00\",\n                \"onset\": \"2025-12-03T14:45:00+10:00\",\n                \"expires\": \"2025-12-04T04:00:00+10:00\",\n                \"ends\": \"2025-12-04T04:00:00+10:00\",\n                \"status\": \"Actual\",\n                \"messageType\": \"Update\",\n                \"category\": \"Met\",\n                \"severity\": \"Moderate\",\n                \"certainty\": \"Likely\",\n                \"urgency\": \"Expected\",\n                \"event\": \"Rip Current Statement\",\n                \"sender\": \"w-nws.webmaster@noaa.gov\",\n                \"senderName\": \"NWS Tiyan GU\",\n                \"headline\": \"Rip Current Statement issued December 3 at 2:45PM ChST until December 4 at 4:00AM ChST by NWS Tiyan GU\",\n                \"description\": \"* WHAT...Large breaking waves of 7 to 9 feet and dangerous rip\\ncurrents.\\n\\n* WHERE...For the High Surf Advisory, north facing reefs. For the\\nHigh Rip Current Risk, north and east facing reefs.\\n\\n* WHEN...Until 4 AM ChST Thursday.\\n\\n* IMPACTS...Dangerous swimming and surfing conditions and\\nlocalized beach erosion. Rip currents can sweep even the best\\nswimmers away from shore into deeper water.\\n\\n* ADDITIONAL DETAILS...Trade-wind swell and a pulse of long-period\\nnortheast swell are producing hazardous surf along north facing\\nreefs and a high risk of rip currents along north and east\\nfacing reefs. These swells are on a downward trend, however,\\nthey are experiencing pulses of higher swell heights. These\\npulses will gradually weaken evening and overnight hours,\\nallowing the surf and risk of rip currents to fall below the 9\\nfoot criteria levels.\",\n                \"instruction\": \"Rip currents will be life threatening. Inexperienced swimmers\\nshould remain out of the water due to dangerous surf conditions.\\nIf caught in a rip current, relax and float. Don't swim against\\nthe current. If able, swim in a direction following the shoreline.\\nIf unable to escape, face the shore and call or wave for help.\",\n                \"response\": \"Avoid\",\n                \"parameters\": {\n                    \"AWIPSidentifier\": [\n                        \"CFWGUM\"\n                    ],\n                    \"WMOidentifier\": [\n                        \"WHMY40 PGUM 030445\"\n                    ],\n                    \"NWSheadline\": [\n                        \"HIGH SURF ADVISORY REMAINS IN EFFECT UNTIL 4 AM CHST THURSDAY... ...HIGH RIP CURRENT RISK REMAINS IN EFFECT THROUGH LATE TONIGHT\"\n                    ],\n                    \"BLOCKCHANNEL\": [\n                        \"EAS\",\n                        \"NWEM\",\n                        \"CMAS\"\n                    ],\n                    \"VTEC\": [\n                        \"/O.EXT.PGUM.RP.S.0018.000000T0000Z-251203T1800Z/\"\n                    ],\n                    \"eventEndingTime\": [\n                        \"2025-12-04T04:00:00+10:00\"\n                    ],\n                    \"expiredReferences\": [\n                        \"w-nws.webmaster@noaa.gov,urn:oid:2.49.0.1.840.0.e8d89e06d7b7159ea55ce7edf91fce61fb2ae35c.001.2,2025-12-02T03:59:00+10:00 w-nws.webmaster@noaa.gov,urn:oid:2.49.0.1.840.0.72a4921e5d890486ce7be3efaf29f9341ee22edb.001.2,2025-12-01T15:44:00+10:00 w-nws.webmaster@noaa.gov,urn:oid:2.49.0.1.840.0.5a377aeea1b3819e99fb54a0cbed24d8c1f12a09.001.2,2025-12-01T04:35:00+10:00 w-nws.webmaster@noaa.gov,urn:oid:2.49.0.1.840.0.aebe29e1a1042d2452398d14a015e88084b7b435.001.2,2025-11-30T18:50:00+10:00 w-nws.webmaster@noaa.gov,urn:oid:2.49.0.1.840.0.3415960b908d87171db6753ca49c552bc054c308.001.1,2025-11-30T15:54:00+10:00 w-nws.webmaster@noaa.gov,urn:oid:2.49.0.1.840.0.71528f877fb6ec75ab31c30c9a375092b0e3e527.001.1,2025-11-30T05:31:00+10:00 w-nws.webmaster@noaa.gov,urn:oid:2.49.0.1.840.0.83b795d79f0afe073a544a7bc9ed2161cf49b640.001.1,2025-11-29T15:36:00+10:00\"\n                    ]\n                },\n                \"scope\": \"Public\",\n                \"code\": \"IPAWSv1.0\",\n                \"language\": \"en-US\",\n                \"web\": \"http://www.weather.gov\",\n                \"eventCode\": {\n                    \"SAME\": [\n                        \"NWS\"\n                    ],\n                    \"NationalWeatherService\": [\n                        \"RPS\"\n                    ]\n                }\n            }\n        },\n        {\n            \"id\": \"https://api.weather.gov/alerts/urn:oid:2.49.0.1.840.0.f25f3139d57c0fbafce18e4394cec8e3387cc317.001.1\",\n            \"type\": \"Feature\",\n            \"geometry\": null,\n            \"properties\": {\n                \"@id\": \"https://api.weather.gov/alerts/urn:oid:2.49.0.1.840.0.f25f3139d57c0fbafce18e4394cec8e3387cc317.001.1\",\n                \"@type\": \"wx:Alert\",\n                \"id\": \"urn:oid:2.49.0.1.840.0.f25f3139d57c0fbafce18e4394cec8e3387cc317.001.1\",\n                \"areaDesc\": \"Guam; Rota; Tinian; Saipan\",\n                \"geocode\": {\n                    \"SAME\": [\n                        \"066010\",\n                        \"069100\",\n                        \"069120\",\n                        \"069110\"\n                    ],\n                    \"UGC\": [\n                        \"GUZ001\",\n                        \"MPZ001\",\n                        \"MPZ002\",\n                        \"MPZ003\"\n                    ]\n                },\n                \"affectedZones\": [\n                    \"https://api.weather.gov/zones/forecast/GUZ001\",\n                    \"https://api.weather.gov/zones/forecast/MPZ001\",\n                    \"https://api.weather.gov/zones/forecast/MPZ002\",\n                    \"https://api.weather.gov/zones/forecast/MPZ003\"\n                ],\n                \"references\": [\n                    {\n                        \"@id\": \"https://api.weather.gov/alerts/urn:oid:2.49.0.1.840.0.5c24cf00b8ce0d30ec10243f5e3d0d1b92563257.001.1\",\n                        \"identifier\": \"urn:oid:2.49.0.1.840.0.5c24cf00b8ce0d30ec10243f5e3d0d1b92563257.001.1\",\n                        \"sender\": \"w-nws.webmaster@noaa.gov\",\n                        \"sent\": \"2025-12-02T15:11:00+10:00\"\n                    },\n                    {\n                        \"@id\": \"https://api.weather.gov/alerts/urn:oid:2.49.0.1.840.0.56606cf3de3759568a567931443b4c170707798d.001.1\",\n                        \"identifier\": \"urn:oid:2.49.0.1.840.0.56606cf3de3759568a567931443b4c170707798d.001.1\",\n                        \"sender\": \"w-nws.webmaster@noaa.gov\",\n                        \"sent\": \"2025-12-03T04:02:00+10:00\"\n                    }\n                ],\n                \"sent\": \"2025-12-03T14:45:00+10:00\",\n                \"effective\": \"2025-12-03T14:45:00+10:00\",\n                \"onset\": \"2025-12-03T14:45:00+10:00\",\n                \"expires\": \"2025-12-04T04:00:00+10:00\",\n                \"ends\": \"2025-12-04T04:00:00+10:00\",\n                \"status\": \"Actual\",\n                \"messageType\": \"Update\",\n                \"category\": \"Met\",\n                \"severity\": \"Minor\",\n                \"certainty\": \"Likely\",\n                \"urgency\": \"Expected\",\n                \"event\": \"High Surf Advisory\",\n                \"sender\": \"w-nws.webmaster@noaa.gov\",\n                \"senderName\": \"NWS Tiyan GU\",\n                \"headline\": \"High Surf Advisory issued December 3 at 2:45PM ChST until December 4 at 4:00AM ChST by NWS Tiyan GU\",\n                \"description\": \"* WHAT...Large breaking waves of 7 to 9 feet and dangerous rip\\ncurrents.\\n\\n* WHERE...For the High Surf Advisory, north facing reefs. For the\\nHigh Rip Current Risk, north and east facing reefs.\\n\\n* WHEN...Until 4 AM ChST Thursday.\\n\\n* IMPACTS...Dangerous swimming and surfing conditions and\\nlocalized beach erosion. Rip currents can sweep even the best\\nswimmers away from shore into deeper water.\\n\\n* ADDITIONAL DETAILS...Trade-wind swell and a pulse of long-period\\nnortheast swell are producing hazardous surf along north facing\\nreefs and a high risk of rip currents along north and east\\nfacing reefs. These swells are on a downward trend, however,\\nthey are experiencing pulses of higher swell heights. These\\npulses will gradually weaken evening and overnight hours,\\nallowing the surf and risk of rip currents to fall below the 9\\nfoot criteria levels.\",\n                \"instruction\": \"Rip currents will be life threatening. Inexperienced swimmers\\nshould remain out of the water due to dangerous surf conditions.\\nIf caught in a rip current, relax and float. Don't swim against\\nthe current. If able, swim in a direction following the shoreline.\\nIf unable to escape, face the shore and call or wave for help.\",\n                \"response\": \"Avoid\",\n                \"parameters\": {\n                    \"AWIPSidentifier\": [\n                        \"CFWGUM\"\n                    ],\n                    \"WMOidentifier\": [\n                        \"WHMY40 PGUM 030445\"\n                    ],\n                    \"NWSheadline\": [\n                        \"HIGH SURF ADVISORY REMAINS IN EFFECT UNTIL 4 AM CHST THURSDAY... ...HIGH RIP CURRENT RISK REMAINS IN EFFECT THROUGH LATE TONIGHT\"\n                    ],\n                    \"BLOCKCHANNEL\": [\n                        \"EAS\",\n                        \"NWEM\",\n                        \"CMAS\"\n                    ],\n                    \"VTEC\": [\n                        \"/O.EXT.PGUM.SU.Y.0037.000000T0000Z-251203T1800Z/\"\n                    ],\n                    \"eventEndingTime\": [\n                        \"2025-12-04T04:00:00+10:00\"\n                    ],\n                    \"expiredReferences\": [\n                        \"w-nws.webmaster@noaa.gov,urn:oid:2.49.0.1.840.0.e8d89e06d7b7159ea55ce7edf91fce61fb2ae35c.001.1,2025-12-02T03:59:00+10:00 w-nws.webmaster@noaa.gov,urn:oid:2.49.0.1.840.0.72a4921e5d890486ce7be3efaf29f9341ee22edb.001.1,2025-12-01T15:44:00+10:00 w-nws.webmaster@noaa.gov,urn:oid:2.49.0.1.840.0.5a377aeea1b3819e99fb54a0cbed24d8c1f12a09.001.1,2025-12-01T04:35:00+10:00 w-nws.webmaster@noaa.gov,urn:oid:2.49.0.1.840.0.aebe29e1a1042d2452398d14a015e88084b7b435.001.1,2025-11-30T18:50:00+10:00\"\n                    ]\n                },\n                \"scope\": \"Public\",\n                \"code\": \"IPAWSv1.0\",\n                \"language\": \"en-US\",\n                \"web\": \"http://www.weather.gov\",\n                \"eventCode\": {\n                    \"SAME\": [\n                        \"NWS\"\n                    ],\n                    \"NationalWeatherService\": [\n      
